vi "Command Drive Time.vi"(2 "Robot System Functions In":T1, 3 "Startup":bool, 4 "String Parameter":string, 5 "Cmd Parameter 3":dbl, 6 "Cmd Parameter 2":dbl, 7 "Cmd Parameter 1":dbl) -> (0 "Robot System Functions Out":T1, 1 "Completed":bool)   [LabVIEW 2016]
uses:
  Subsystems/All Robot Commands.ctl
  Subsystems/Drive and Climb SS/Drive + Climb Commands 2017.ctl
  Subsystems/Gear Delivery SS/Gear Delivery Commands.ctl
  Subsystems/Conveyor and Shooter SS/Conveyor and Shooter Commands.ctl
  Subsystems/Ball Intake SS/Ball Intake Commands.ctl
  Command Execution State.ctl
  <vilib>/Rock Robotics/WPI/ThirdParty/CanMotor/TalonSRX/WPI_CANTalonSRX_APIControlMode.ctl
  Global Variables/Refnum Names.vi
  Global Variables/Auto Drive Calibrations.vi
panel:
  out "Right F":dbl
  out "Right D":dbl
  out "Right I":dbl
  out "Right P":dbl
  out "Left F":dbl
  out "Left D":dbl
  out "Left I":dbl
  out "Left P":dbl
  # "Sample robot\ncontrol output.\nReplace with \nactual teleop \ncontrol signal \nstructure."
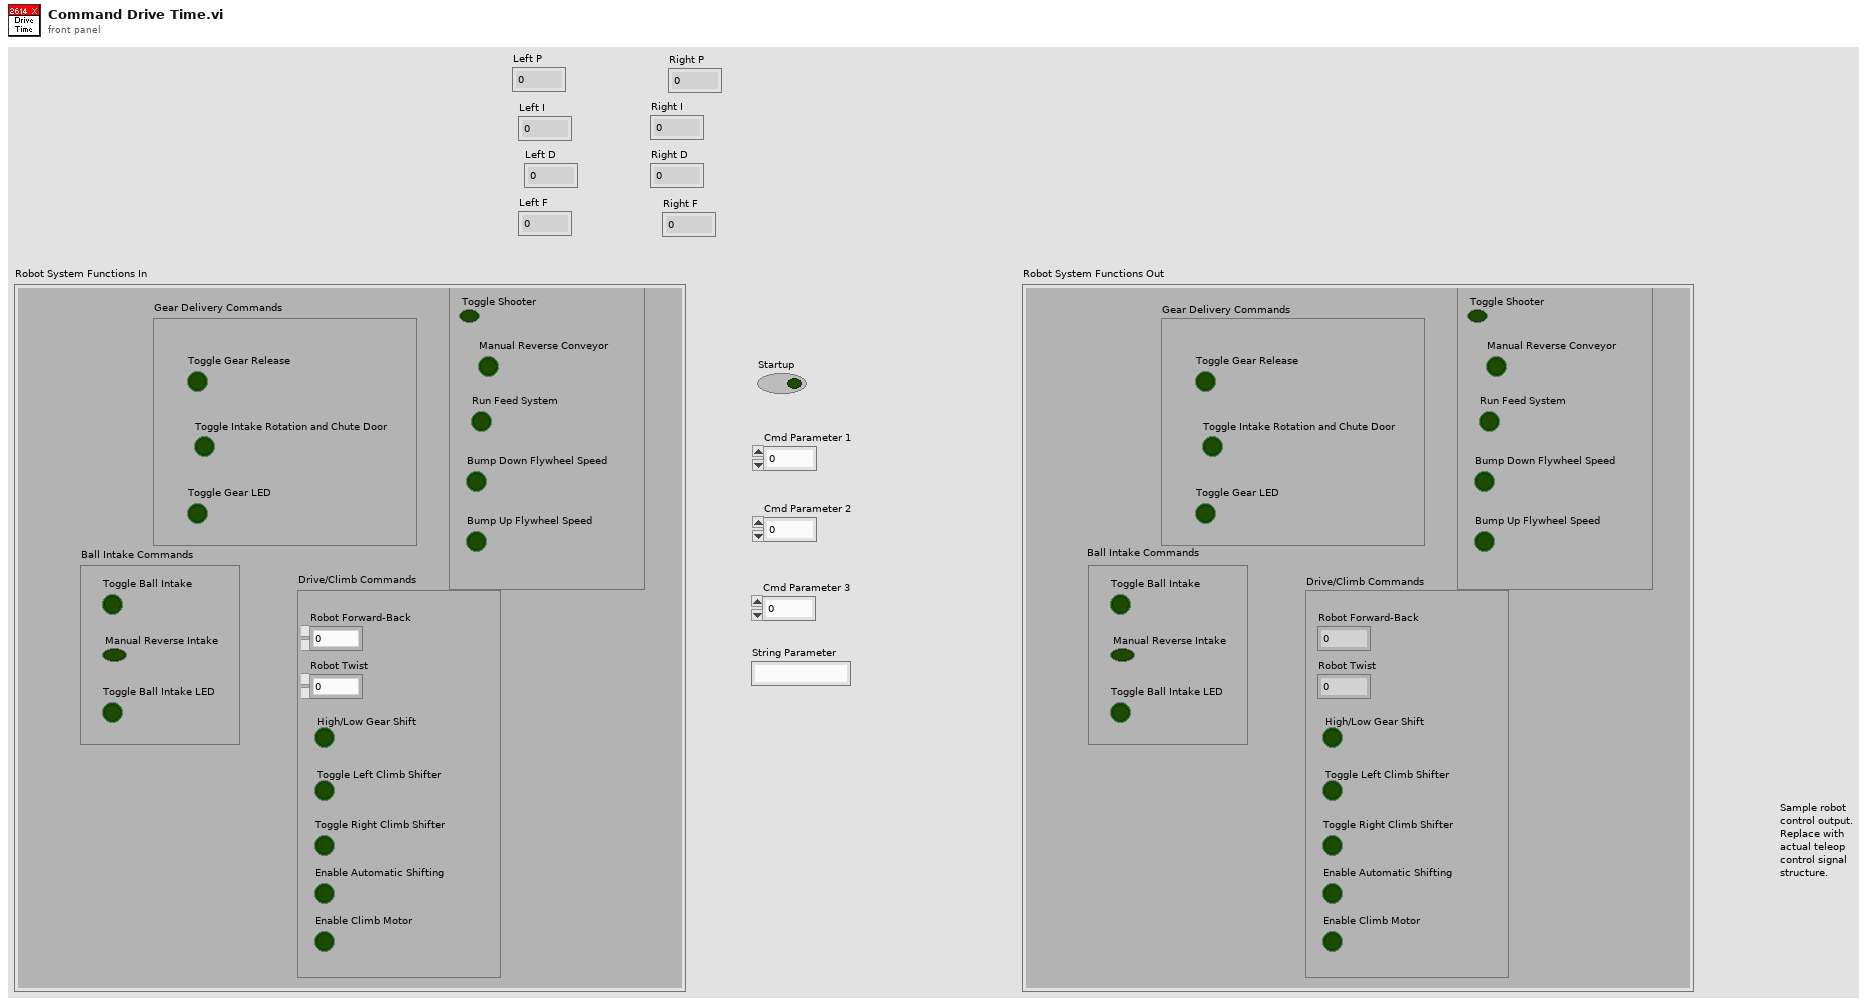
[diagram p1: front panel]
types:
  T1 = typedef "All Robot Commands.ctl" = cluster{"Drive/Climb Commands":T2, "Gear Delivery Commands":T3, "Shooter and Conveyor Commands":T4, "Ball Intake Commands":T5}
  T2 = typedef "Drive + Climb Commands 2017.ctl" = cluster{"Robot Forward-Back":dbl, "Robot Twist":dbl, "High/Low Gear Shift":bool, "Toggle Left Climb Shifter":bool, "Toggle Right Climb Shifter":bool, "Enable Automatic Shifting":bool, "Enable Climb Motor ":bool}
  T3 = typedef "Gear Delivery Commands.ctl" = cluster{"Toggle Gear Release":bool, "Toggle Intake Rotation and Chute Door":bool, "Toggle Gear LED":bool}
  T4 = typedef "Conveyor and Shooter Commands.ctl" = cluster{"Toggle Shooter":bool, "Manual Reverse Conveyor":bool, "Run Feed System":bool, "Bump Down Flywheel Speed":bool, "Bump Up Flywheel Speed":bool}
  T5 = typedef "Ball Intake Commands.ctl" = cluster{"Toggle Ball Intake":bool, "Manual Reverse Intake":bool, "Toggle Ball Intake LED":bool}
  T6 = typedef "Command Execution State.ctl" = enum16{"Initialize", "Execute", "Finish"}
  T7 = typedef "WPI_CANTalonSRX_APIControlMode.ctl" = enum8{"Percent VBus", "Speed", "Position", "Slave", "Unchanged / Invalid", "Voltage Compensation", "Current", "Motion Profile", "Motion Magic"}
  T8 = typedef "WPI_MotorControlDeviceRef.ctl" = cluster{"DeviceStatus":errorcluster, "Type":T9, "PWM":cluster{"PWM Channel":T10, "DeadBand":T11}, "CAN":cluster{"Device Number":u8, "SetOutput VI Ref":variant, "GetOutput VI Ref":variant, "Enable VI Ref":variant, "Disable VI Ref":variant, "Data":variant}, "Invert":bool}
  T9 = typedef "WPI_MotorControlType.ctl" = enum16{"PWM", "CAN"}
  T10 = typedef "FPGA_DIOPWMChannel.ctl" = enum8{"PWM 0", "PWM 1", "PWM 2", "PWM 3", "PWM 4", "PWM 5", "PWM 6", "PWM 7", "PWM 8", "PWM 9", "PWM MXP 0", "PWM MXP 1", "PWM MXP 2", "PWM MXP 3", "PWM MXP 4", "PWM MXP 5", "PWM MXP 6", "PWM MXP 7", "PWM MXP 8", "PWM MXP 9", "Invalid"}
  T11 = typedef "WPI_PWMDeadband.ctl" = cluster{"Name":string, "maxPositivePwm":i32, "minPositivePwm":i32, "centerPwm":i32, "maxNegativePwm":i32, "minNegativePwm":i32, "angularRange":u16}
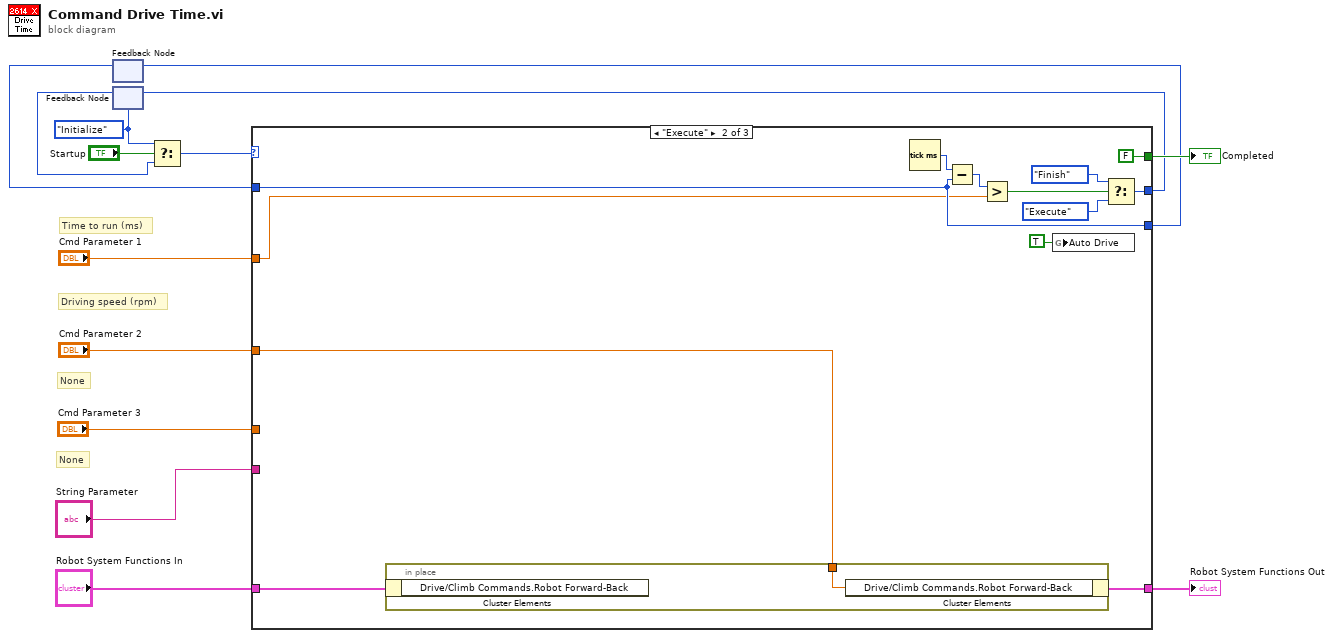
[diagram p0: block diagram]
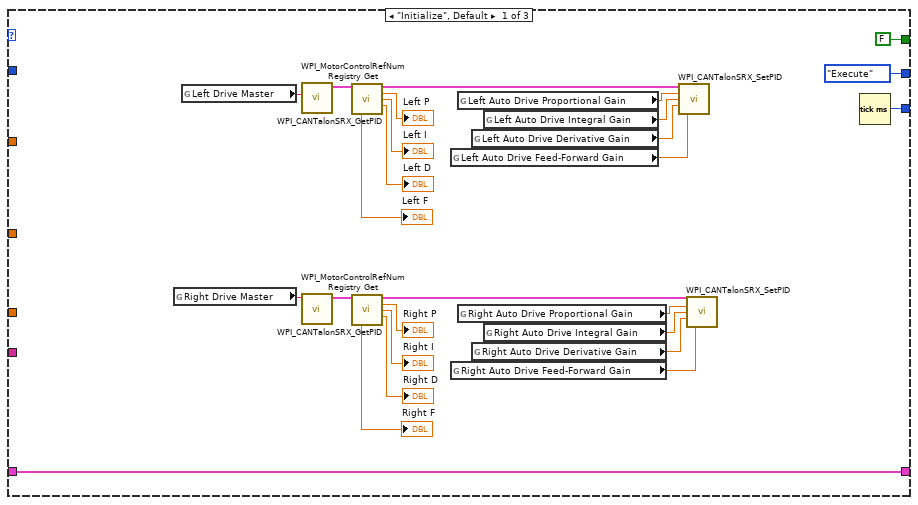
[diagram p2: hidden frame]
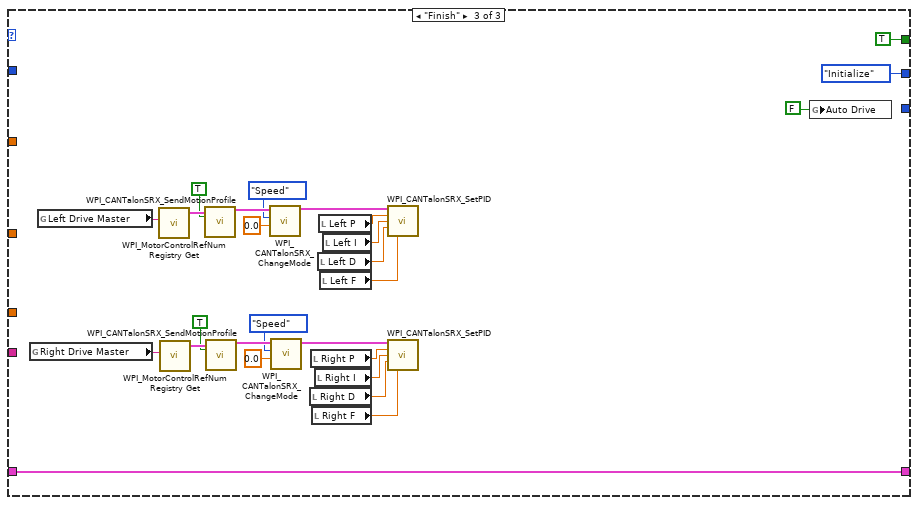
[diagram p3: hidden frame]
diagram:
  w9 = Command_Execution_State."Initialize" ("Play State")
  # "None"
  # "None"
  # "Driving speed (rpm)"
  # "Time to run (ms)"
  n1 = feedback #1() -> (w1:u32)  [unwired: 1 in]
  n2 = feedback #2(w9) -> (w10:T6)
  n3 = Select(t=w9, s="Startup", f=w10) -> (s? t:f=w14:T6)
  n4 = case shown="\"Execute\"" w14 {
    tunnel: [FALSE FALSE TRUE] -> w12
    tunnel: [Command_Execution_State."Execute" ("Play State") w51 Command_Execution_State."Initialize" ("f")] -> w11
    tunnel: "Cmd Parameter 1" -> [_ w45 _]
    tunnel: "Cmd Parameter 2" -> [_ w43 _]
    tunnel: [w38 w42 w78] -> w6
    tunnel: "Robot System Functions In" -> [w38 w49 w78]
    tunnel: "Cmd Parameter 3" -> [_ _ _]
    tunnel: "String Parameter" -> [_ _ _]
    tunnel: [w37 w47 _] -> w2
    tunnel: w1 -> [_ w47 _]
    frame "Initialize", Default {
      n5 = global read "Refnum Names.vi" "Right Drive Master"() -> (w30:string)
      n6 = global read "Refnum Names.vi" "Left Drive Master"() -> (w36:string)
      n7 = call <vilib>:"WPI_MotorControlRefNum Registry Get.vi"("refnum name"=w36) -> ("MotorControlDevRef"=w35:T8)  [unwired: 9 in, 1 out]
      n8 = call <vilib>:"WPI_MotorControlRefNum Registry Get.vi"("refnum name"=w30) -> ("MotorControlDevRef"=w29:T8)  [unwired: 9 in, 1 out]
      n9 = call <vilib>:"WPI_CANTalonSRX_GetPID.vi"("CAN Talon SRX Ref"=w35) -> ("CAN Talon SRX Ref"=w16:T8, "P"=→"Left P":dbl, "I"=→"Left I":dbl, "D"=→"Left D":dbl, "F"=→"Left F":dbl)  [unwired: 7 in, 3 out]
      n10 = call <vilib>:"WPI_CANTalonSRX_GetPID.vi"("CAN Talon SRX Ref"=w29) -> ("CAN Talon SRX Ref"=w15:T8, "P"=→"Right P":dbl, "I"=→"Right I":dbl, "D"=→"Right D":dbl, "F"=→"Right F":dbl)  [unwired: 7 in, 3 out]
      n11 = global read "Auto Drive Calibrations.vi" "Left Auto Drive Feed-Forward Gain"() -> (w17:dbl)
      n12 = global read "Auto Drive Calibrations.vi" "Right Auto Drive Feed-Forward Gain"() -> (w22:dbl)
      n13 = global read "Auto Drive Calibrations.vi" "Left Auto Drive Proportional Gain"() -> (w20:dbl)
      n14 = global read "Auto Drive Calibrations.vi" "Right Auto Drive Proportional Gain"() -> (w21:dbl)
      n15 = global read "Auto Drive Calibrations.vi" "Left Auto Drive Derivative Gain"() -> (w18:dbl)
      n16 = global read "Auto Drive Calibrations.vi" "Right Auto Drive Derivative Gain"() -> (w23:dbl)
      n17 = global read "Auto Drive Calibrations.vi" "Left Auto Drive Integral Gain"() -> (w19:dbl)
      n18 = global read "Auto Drive Calibrations.vi" "Right Auto Drive Integral Gain"() -> (w24:dbl)
      n19 = call <vilib>:"WPI_CANTalonSRX_SetPID.vi"("CAN Talon SRX Ref"=w16, "P"=w20, "I"=w19, "D"=w18, "F"=w17) -> ()  [unwired: 9 in, 2 out]
      n20 = call <vilib>:"WPI_CANTalonSRX_SetPID.vi"("CAN Talon SRX Ref"=w15, "P"=w21, "I"=w24, "D"=w23, "F"=w22) -> ()  [unwired: 9 in, 2 out]
      n21 = Tick Count (ms)() -> (millisecond timer value=w37:u32)
    }
    frame "Execute" {
      n22 = in-place {
        in-place-border: w43 -> [w54]
        n23 = in-place-cluster #3(w49) -> ()  [unwired: 1 out]
        n24 = in-place-cluster #3("Drive/Climb Commands.Robot Forward-Back"=w54) -> (w42:T1)
      }
      n25 = Tick Count (ms)() -> (millisecond timer value=w48:u32)
      n26 = Subtract(x=w48, y=w47) -> (x-y=w46:u32)
      n27 = Greater?(x=w46, y=w45) -> (0:w44:bool)
      n28 = global write "Auto Drive Calibrations.vi" "Auto Drive"(TRUE ("PID Heading")) -> ()
      n29 = Select(t=Command_Execution_State."Finish" ("Play State"), s=w44, f=Command_Execution_State."Execute") -> (s? t:f=w51:T6)
    }
    frame "Finish" {
      n30 = global read "Refnum Names.vi" "Right Drive Master"() -> (w56:string)
      n31 = global read "Refnum Names.vi" "Left Drive Master"() -> (w68:string)
      n32 = call <vilib>:"WPI_MotorControlRefNum Registry Get.vi"("refnum name"=w68) -> ("MotorControlDevRef"=w73:T8)  [unwired: 9 in, 1 out]
      n33 = call <vilib>:"WPI_MotorControlRefNum Registry Get.vi"("refnum name"=w56) -> ("MotorControlDevRef"=w61:T8)  [unwired: 9 in, 1 out]
      n34 = call <vilib>:"WPI_CANTalonSRX_SendMotionProfile.vi"("CAN Talon SRX Ref"=w73, "Clear"=TRUE) -> ("CAN Talon SRX Ref Out"=w70:T8)  [unwired: 10 in, 3 out]
      n35 = call <vilib>:"WPI_CANTalonSRX_SendMotionProfile.vi"("CAN Talon SRX Ref"=w61, "Clear"=TRUE) -> ("CAN Talon SRX Ref Out"=w58:T8)  [unwired: 10 in, 3 out]
      n36 = call <vilib>:"WPI_CANTalonSRX_ChangeMode.vi"("Output"=0.0, "Control Mode"=WPI_CANTalonSRX_APIControlMode."Speed", "CAN Talon SRX Ref"=w70) -> ("CAN Talon SRX Ref"=w67:T8)  [unwired: 7 in, 1 out]
      n37 = call <vilib>:"WPI_CANTalonSRX_ChangeMode.vi"("Output"=0.0, "Control Mode"=WPI_CANTalonSRX_APIControlMode."Speed", "CAN Talon SRX Ref"=w58) -> ("CAN Talon SRX Ref"=w55:T8)  [unwired: 7 in, 1 out]
      n38 = local read "Right D"() -> (w75:dbl)
      n39 = local read "Right P"() -> (w77:dbl)
      n40 = local read "Right F"() -> (w74:dbl)
      n41 = local read "Right I"() -> (w76:dbl)
      n42 = local read "Left D"() -> (w64:dbl)
      n43 = local read "Left P"() -> (w66:dbl)
      n44 = local read "Left F"() -> (w63:dbl)
      n45 = local read "Left I"() -> (w65:dbl)
      n46 = call <vilib>:"WPI_CANTalonSRX_SetPID.vi"("CAN Talon SRX Ref"=w67, "P"=w66, "I"=w65, "D"=w64, "F"=w63) -> ()  [unwired: 9 in, 2 out]
      n47 = call <vilib>:"WPI_CANTalonSRX_SetPID.vi"("CAN Talon SRX Ref"=w55, "P"=w77, "I"=w76, "D"=w75, "F"=w74) -> ()  [unwired: 9 in, 2 out]
      n48 = global write "Auto Drive Calibrations.vi" "Auto Drive"(FALSE ("PID Heading")) -> ()
    }
  }
  "Completed" <- w12
  "Robot System Functions Out" <- w6
  n49 = feedback-in #1(w2) -> ()
  n50 = feedback-in #2(w11) -> ()
